vi "Read Test Interval.vi"(8 "error in (no error)":errorcluster, 11 "bt_Parallel_Threaded in":refnum<class "bt_Parallel_Threaded.lvclass">) -> (0 "error out":errorcluster, 2 "Check Interval":u32, 3 "bt_Parallel_Threaded out":refnum<class "bt_Parallel_Threaded.lvclass">)   [LabVIEW 2021, in "BT.lvlib" / "bt_Parallel_Threaded.lvclass"]
uses:
  bt_Parallel_Threaded.lvclass
  bt_Parallel_Threaded.lvclass/bt_Parallel_Threaded.ctl
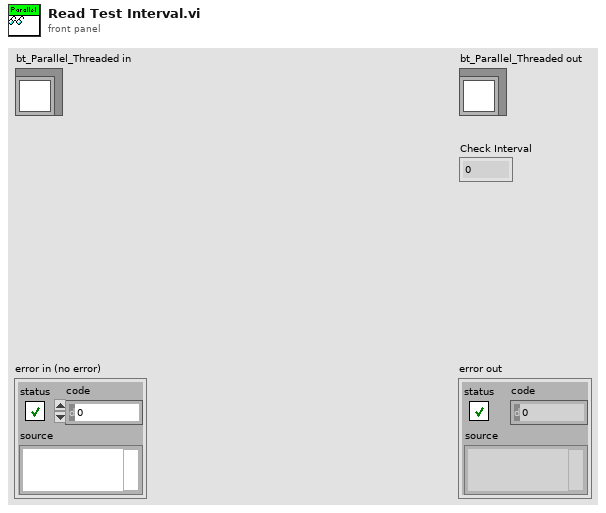
[diagram p1: front panel]
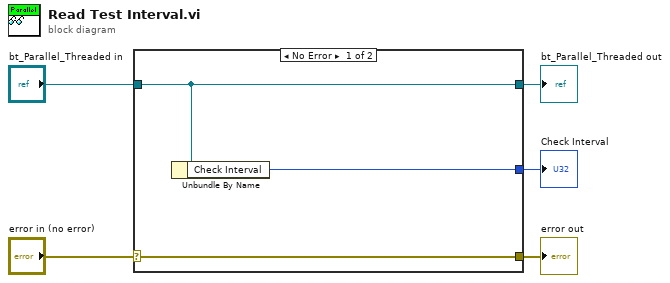
[diagram p0: block diagram]
diagram:
  n1 = case shown="No Error" "error in (no error)" {
    selector: "error in (no error)" -> [w8 w9]
    tunnel: [w8 w9] -> w4
    tunnel: [w7 w10] -> w2
    tunnel: "bt_Parallel_Threaded in" -> [w7 w10]
    tunnel: [w6 _] -> w1
    frame No Error {
      n2 = Unbundle By Name(w7) -> ("Check Interval"=w6:i32)
    }
    frame Error {
    }
  }
  "error out" <- w4
  "bt_Parallel_Threaded out" <- w2
  "Check Interval" <- w1
